vi "ReadPart.vi"(7 "number of inputs (Defaut: 60)":u16, 8 "error in (no error)":errorcluster, 9 "starting address (Default: 1)":u16, 10 "Numeric in":dbl, 11 "Modbus Master in":refnum<class "Modbus Master.lvclass">) -> (0 "error out":errorcluster, 2 "Numeric out":dbl, 3 "Modbus Master out":refnum<class "Modbus Master.lvclass">)   [LabVIEW 2019]
uses:
  <vilib>/NI/Modbus Library/API/Master/Modbus Master.lvclass
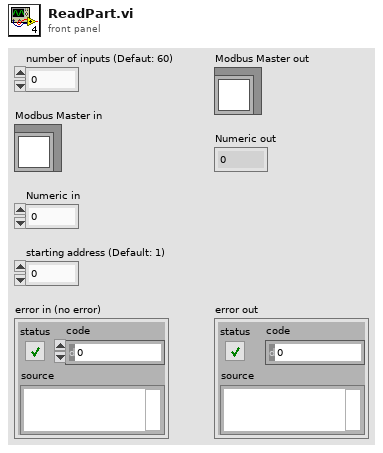
[diagram p1: front panel]
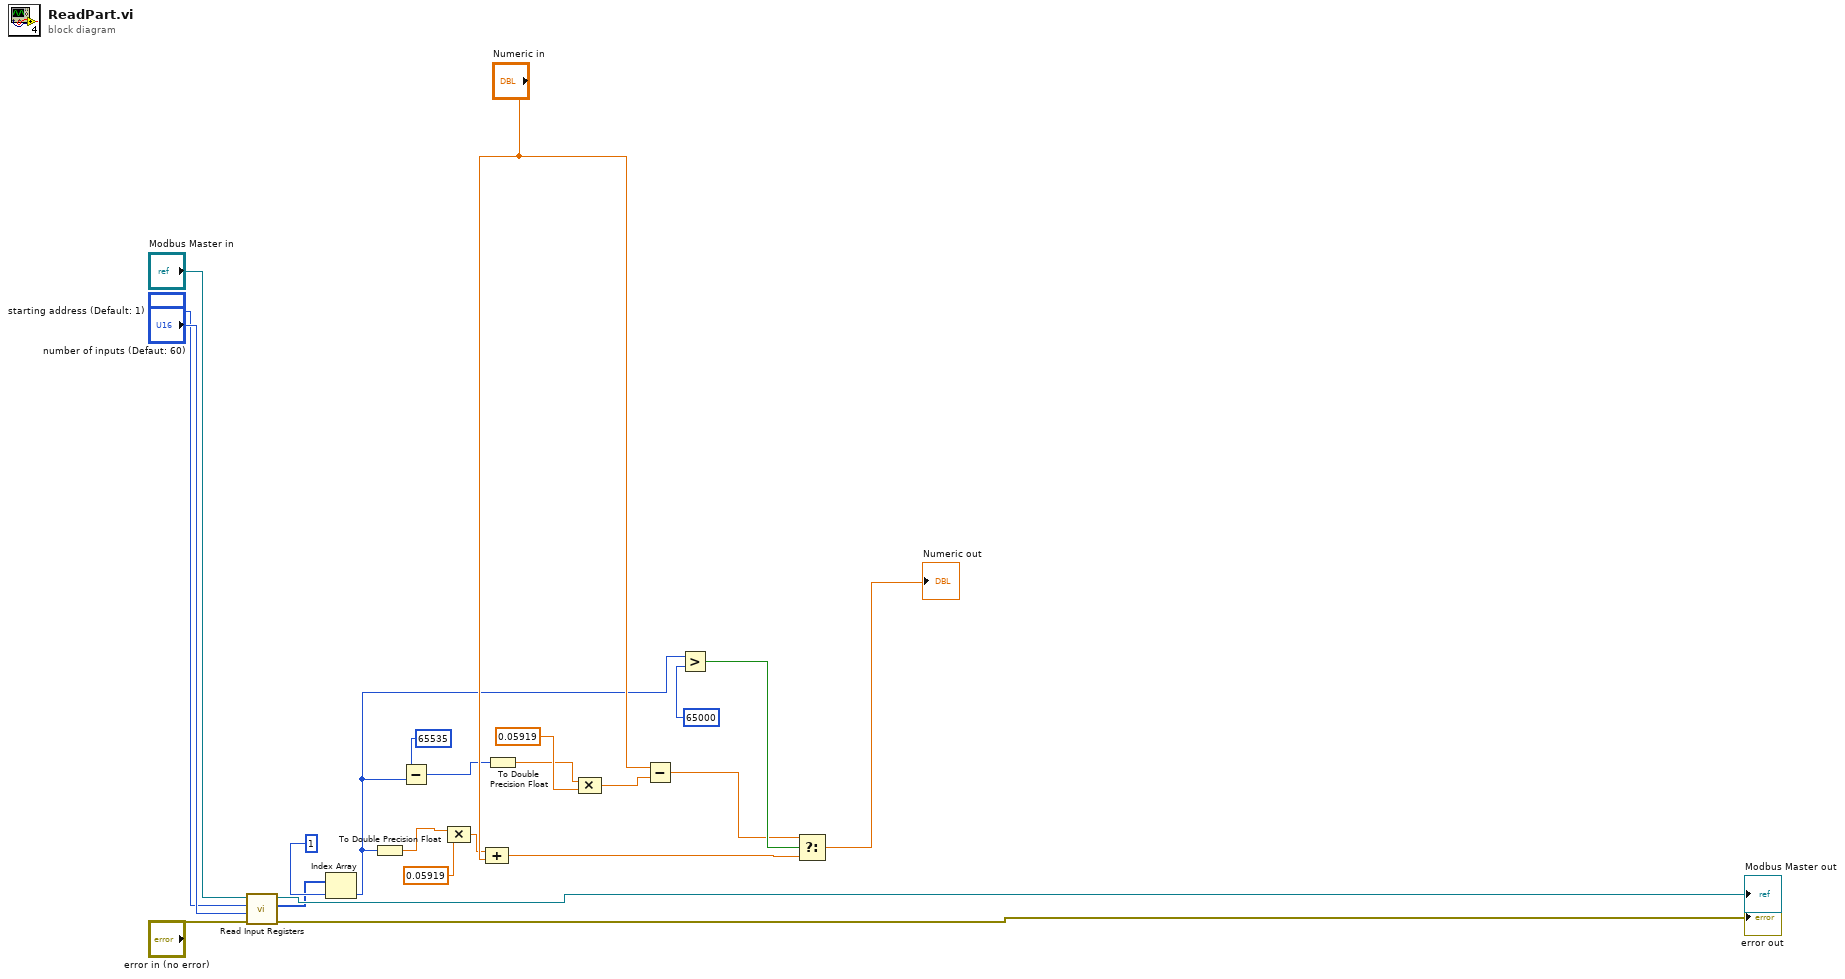
[diagram p0: block diagram]
diagram:
  n1 = call-dynamic "Read Input Registers.vi"("error in"="error in (no error)", "number of inputs"="number of inputs (Defaut: 60)", "starting address"="starting address (Default: 1)", "Modbus master in"="Modbus Master in") -> ("error out"=→"error out":errorcluster, "register values"=w1:u16[], "Modbus master out"=→"Modbus Master out":refnum<class "Modbus Master.lvclass">)  [unwired: 5 in]
  n2 = Index Array(array=w1, index=1) -> (element=w10:u16)
  n3 = To Double Precision Float(number=w10) -> (double precision float=w6:dbl)
  n4 = Subtract(x=u16 65535 ("y"), y=w10) -> (x-y=w14:u16)
  n5 = Compound Arithmetic op=MULTIPLY(w6, 0.05919 ("value")) -> (w3:dbl)
  n6 = Compound Arithmetic op=ADD(w3, "Numeric in") -> (w17:dbl)
  n7 = To Double Precision Float(number=w14) -> (double precision float=w12:dbl)
  n8 = Compound Arithmetic op=MULTIPLY(w12, 0.05919 ("value")) -> (w15:dbl)
  n9 = Subtract(x="Numeric in", y=w15) -> (x-y=w16:dbl)
  n10 = Greater?(x=w10, y=u16 65000) -> (0:w18:bool)
  n11 = Select(t=w16, s=w18, f=w17) -> (s? t:f=→"Numeric out":dbl)
